vi "create tag.vi"(6 "raw default":string, 7 "metadata":string, 8 "error in":errorcluster, 9 "data type":T1, 10 "name":string, 11 "tag descriptor in":refnum<class "tag descriptor.lvclass">) -> (0 "error out":errorcluster, 3 "tag descriptor out":refnum<class "tag descriptor.lvclass">)   [LabVIEW 2013, in "tag bus.lvlib" / "tag descriptor.lvclass"]
uses:
  tag descriptor.lvclass
  Data Type.ctl
  tag descriptor.lvclass/tag descriptor.ctl
  tag bus.lvlib
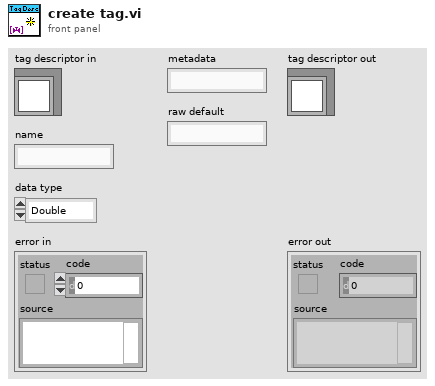
[diagram p1: front panel]
types:
  T1 = typedef "tag bus.lvlib/tag descriptor.lvclass/Data Type.ctl" = enum16{"Double", "Single", "I64", "I32", "I16", "I8", "U64", "U32", "U16", "U8", "Boolean", "String", "Array of Double", "Array of Single", "Array of I64", "Array of I32", "Array of I16", "Array of I8", "Array of U64", "Array of U32", "Array of U16", "Array of U8", "Array of Boolean", "Array of String"}
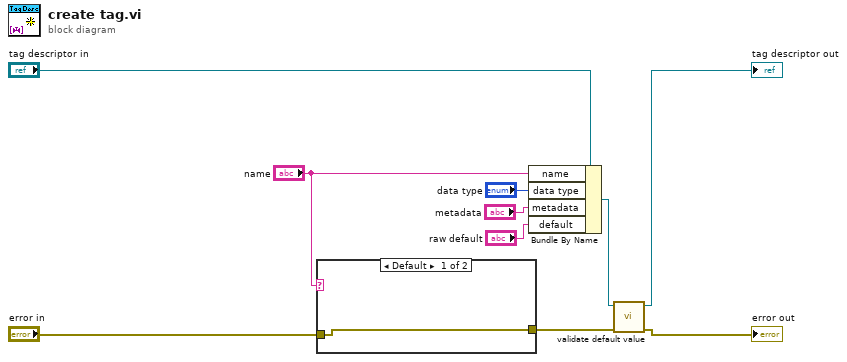
[diagram p0: block diagram]
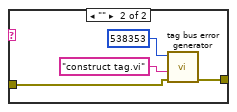
[diagram p2: hidden frame]
diagram:
  n1 = case shown="Default" "name" {
    tunnel: [w11 w15] -> w6
    tunnel: "error in" -> [w11 w12]
    frame Default {
    }
    frame "" {
      n2 = call "tag bus error generator.vi"("error in"=w12, "source"="construct tag.vi", "error code (0)"=538353) -> ("error out"=w15:errorcluster)  [unwired: 6 in]
    }
  }
  n3 = Bundle By Name(cluster="tag descriptor in", "name"="name", "data type"="data type", "metadata"="metadata", "default"="raw default") -> (w5:refnum<class "tag descriptor.lvclass">)
  n4 = call "validate default value.vi"("error in"=w6, "tag descriptor in"=w5) -> ("error out"=→"error out":errorcluster, "tag descriptor out"=→"tag descriptor out":refnum<class "tag descriptor.lvclass">)  [unwired: 7 in, 1 out]
